vi "Page_Info_Write.vi"(6 "ctlReferences":T1, 8 "error in (no error)":errorcluster, 10 "Target filename":string, 11 "AB_EXE in":refnum<class "AB_EXE.lvclass">) -> (0 "error out":errorcluster, 3 "AB_EXE out":refnum<class "AB_EXE.lvclass">)   [LabVIEW 2020, in "AB_EXE.lvclass"]
uses:
  <vilib>/AppBuilder/AB_Classes/EXE/AB_EXE.lvclass
  e:/builds/penguin/labview/branches/2020/dev/dist/vi.lib/AppBuilder/AB_Classes/TargetFile/AB_Targetfile.lvclass
  <resource>/Framework/Providers/Builds/AppBuilder/AB_UI_Page_Info_References.ctl
  <vilib>/AppBuilder/AB_Classes/EXE/AB_EXE.lvclass/AB_EXE.ctl
  <vilib>/AppBuilder/AB_Classes/Application/AB_Application.lvclass
  <vilib>/AppBuilder/AB_Classes/TargetFile/AB_Targetfile.lvclass
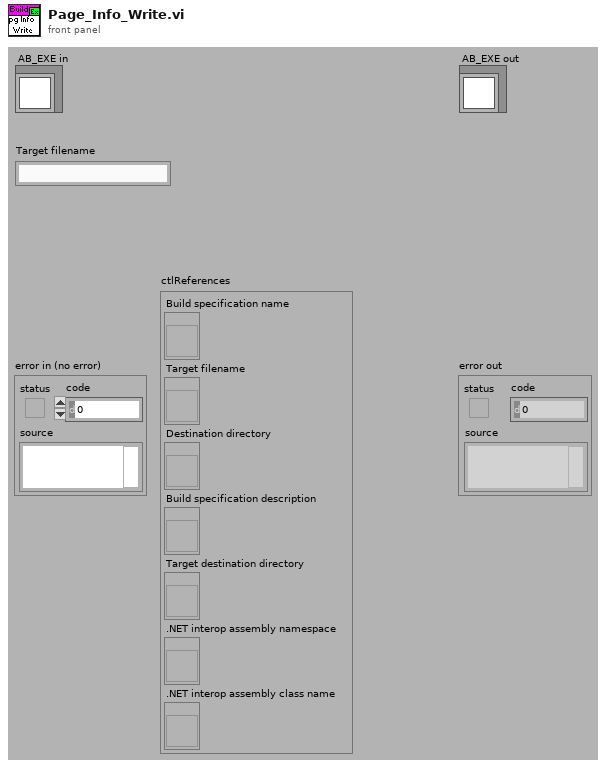
[diagram p1: front panel]
types:
  T1 = typedef "AB_UI_Page_Info_References.ctl" = cluster{"Build specification name":refnum<vi>, "Target filename":refnum<vi>, "Destination directory":refnum<vi>, "Build specification description":refnum<vi>, "Target destination directory":refnum<vi>, ".NET interop assembly namespace":refnum<vi>, ".NET interop assembly class name":refnum<vi>}
  T2 = typedef "AB_Targetfile.ctl" = cluster{"targetfileName":string, "targetfileGUID":string, "enableDebugging":bool, "versionInfo":cluster{"productName":string, "legalCopyright":string, "companyName":string, "internalName":string, "fileDescription":string}, "eng_consolidatedTypeInfo":string, "fastFileFormat":bool, "eng_LEIFBuildData":u32, "versionIndependent":bool}
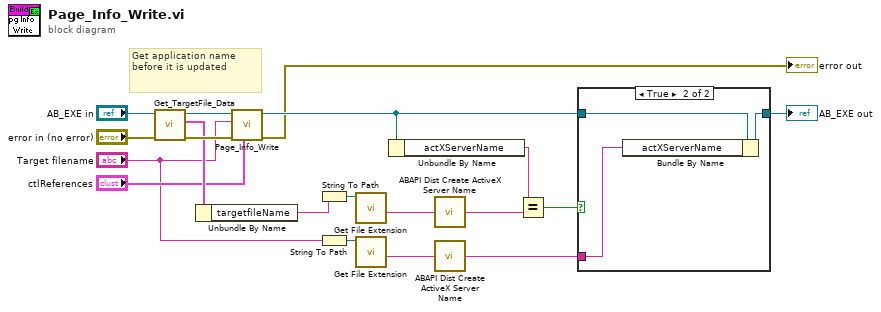
[diagram p0: block diagram]
diagram:
  # "Get application name before it is updated"
  n1 = call <vilib>:"Get_TargetFile_Data.vi"("error in (no error)"="error in (no error)", "AB_Targetfile in"="AB_EXE in") -> ("error out"=w16:errorcluster, "data"=w15:T2, "AB_Targetfile out"=w18:refnum<class "AB_EXE.lvclass">)  [unwired: 7 in]
  n2 = Unbundle By Name(w15) -> ("targetfileName"=w3:string)
  n3 = call-parent "Page_Info_Write.vi"("ctlReferences"="ctlReferences", "error in (no error)"=w16, "Target filename"="Target filename", "AB_Targetfile in"=w18) -> ("error out"=→"error out":errorcluster, "AB_Targetfile out"=w10:refnum<class "AB_EXE.lvclass">)  [unwired: 6 out]
  n4 = String To Path(string=w3) -> (path=w6:path)
  n5 = String To Path(string="Target filename") -> (path=w5:path)
  n6 = call <vilib>:"Get File Extension.vi"("file"=w6) -> ("filename without extension"=w2:string)  [unwired: 1 in, 9 out]
  n7 = call <vilib>:"Get File Extension.vi"("file"=w5) -> ("filename without extension"=w4:string)  [unwired: 1 in, 9 out]
  n8 = Unbundle By Name(w10) -> ("actXServerName"=w11:string)
  n9 = call <vilib>:"ABAPI Dist Create ActiveX Server Name.vi"("name"=w2) -> ("activex name"=w14:string)
  n10 = call <vilib>:"ABAPI Dist Create ActiveX Server Name.vi"("name"=w4) -> ("activex name"=w12:string)
  n11 = Equal?(x=w11, y=w14) -> (x = y?=w13:bool)
  n12 = case shown="True" w13 {
    tunnel: w12 -> [_ w23]
    tunnel: w10 -> [w20 w22]
    tunnel: [w20 w21] -> w9
    frame False {
    }
    frame True {
      n13 = Bundle By Name(cluster=w22, "actXServerName"=w23) -> (w21:refnum<class "AB_EXE.lvclass">)
    }
  }
  "AB_EXE out" <- w9
